vi "CameraGetData.vi"(8 "error in (no error)":errorcluster, 10 "keep open?":bool, 11 "AndorSDK2 in":refnum<class "Andor2.lvclass">) -> (0 "error out":errorcluster, 2 "image_data":u16[][][](array[numeric]), 3 "AndorSDK2 out":refnum<class "Andor2.lvclass">)   [LabVIEW 2010, in "Andor2.lvclass"]
uses:
  <userlib>/BIAS2/classes/Andor2/Andor2.lvclass
  <userlib>/BIAS2/classes/Andor2/Andor2.lvclass/Andor2.ctl
  <userlib>/Andor/atmcd32d.llb/Shutter_mode typedef.ctl
  <userlib>/Andor/atmcd32d.llb/Shutter_type typedef.ctl
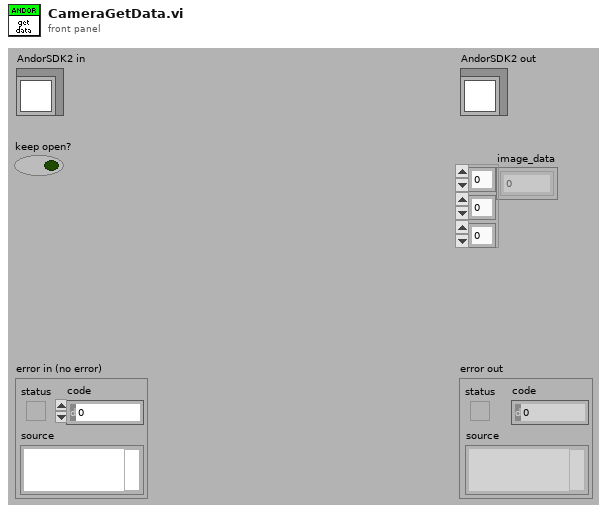
[diagram p1: front panel]
types:
  T1 = typedef "Shutter_mode typedef.ctl" = enum16{"Auto", "Open", "Close"}
  T2 = typedef "Shutter_type typedef.ctl" = enum16{"TTL Low", "TTL High"}
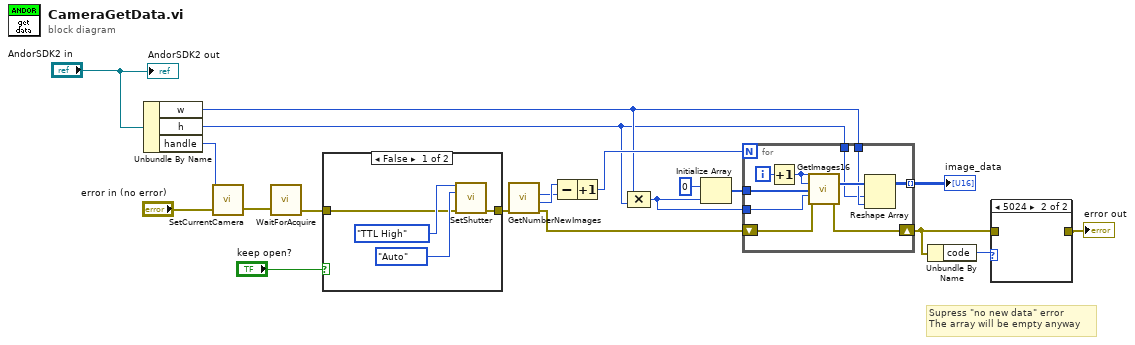
[diagram p0: block diagram]
diagram:
  # "Supress \"no new data\" error\nThe array will be empty anyway"
  n1 = Unbundle By Name("AndorSDK2 in") -> ("w"=w7:i32, "h"=w6:i32, "handle"=w17:i32)
  n2 = call <userlib>:"SetCurrentCamera.vi"("error in (no error)"="error in (no error)", "cameraHandle"=w17) -> ("error out"=w14:errorcluster)  [unwired: 1 out]
  n3 = call <userlib>:"WaitForAcquire.vi"("error in"=w14) -> ("error out"=w15:errorcluster)  [unwired: 2 in, 2 out]
  n4 = case shown="False" "keep open?" {
    tunnel: [w25 w26] -> w5
    tunnel: w15 -> [w22 w26]
    frame False {
      n5 = call <userlib>:"SetShutter.vi"("type"=Shutter_type_typedef."TTL High", "mode"=Shutter_mode_typedef."Auto", "error in (no error)"=w22) -> ("error out"=w25:errorcluster)  [unwired: 11 in, 1 out]
    }
    frame True {
    }
  }
  n6 = call <userlib>:"GetNumberNewImages.vi"("error in (no error)"=w5) -> ("error out"=w9:errorcluster, "last"=w20:i32, "first"=w16:u32)  [unwired: 3 in, 1 out]
  n7 = Subtract(x=w20, y=w16) -> (x-y=w21:u32)
  n8 = Increment(x=w21) -> (x+1=w13:u32)
  n9 = Compound Arithmetic op=MULTIPLY(w7, w6) -> (w10:i32)
  n10 = Initialize Array(u16 0 ("element"), w10) -> (w11:u16[])
  n11 = for {
    N: w13 -> [_]
    tunnel: w11 -> [w36]
    tunnel: w10 -> [w35]
    shift-right: [w32] -> w3
    shift-left: w9 -> [w33]
    tunnel: [w30] -> w8 mode=indexing
    tunnel: w7 -> [w29]
    tunnel: w6 -> [w28]
    i -> [w34]
    n12 = Increment(x=w34) -> (x+1=w27:i32)
    n13 = call <userlib>:"GetImages16.vi"("first"=w27, "last"=w27, "array"=w36, "size"=w35, "error in (no error)"=w33) -> ("array"=w31:u16[], "error out"=w32:errorcluster)  [unwired: 6 in, 3 out]
    n14 = Reshape Array(w31, w28, w29) -> (w30:u16[][])
  }
  "image_data" <- w8
  n15 = Unbundle By Name(w3) -> ("code"=w2:i32)
  n16 = case shown="5024" w2 {
    tunnel: [w37 _] -> w1
    tunnel: w3 -> [w37 _]
    frame Default {
    }
    frame 5024 {
    }
  }
  "error out" <- w1
  "AndorSDK2 out" <- "AndorSDK2 in"
